vi "Map IO.vi"(8 "error in (no error)":errorcluster, 9 "Input Array":u8[](array[numeric]), 10 "Output Array":u8[](array[numeric]), 11 "6509 in":refnum<class "6509.lvclass">) -> (0 "error out":errorcluster, 1 "Boolean Array":bool[](array[boolean]), 2 "Bank Array":u8[](array[numeric]), 3 "6509 out":refnum<class "6509.lvclass">)   [LabVIEW 2019, in "6509.lvlib" / "6509.lvclass"]
uses:
  Library/6509.lvclass
  C:/Users/Public/Documents/Development/builds/Instruments/DIG_IO.lvlibp/Library/DIG_IO.lvclass
  builds/Instruments/DIG_IO.lvlibp/Accessors/Read BankDefs.vi
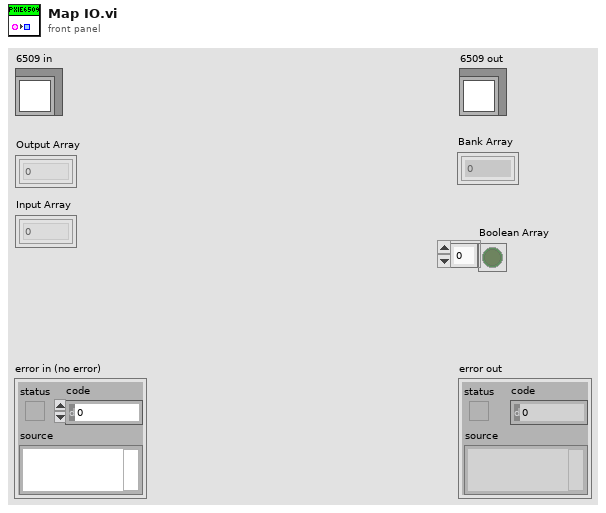
[diagram p1: front panel]
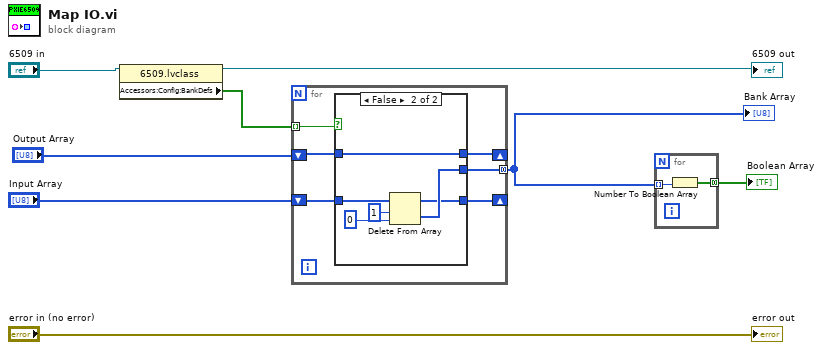
[diagram p0: block diagram]
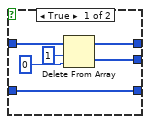
[diagram p2: hidden frame]
diagram:
  n1 = property class="6509.lvclass"(reference="6509 in") -> (reference out=→"6509 out":refnum<class "6509.lvclass">, "Accessors:Config:BankDefs"=w4:bool[])  [unwired: 1 in, 1 out]
  n2 = for {
    tunnel: w4 -> [w14] mode=indexing
    shift-right: [w10] -> _
    shift-left: "Output Array" -> [w13]
    shift-right: [w11] -> _
    shift-left: "Input Array" -> [w12]
    tunnel: [w9] -> w1 mode=concatenating
    n3 = case shown="False" w14 {
      tunnel: w13 -> [w20 w21]
      tunnel: w12 -> [w17 w23]
      tunnel: [w17 w22] -> w11
      tunnel: [w16 w21] -> w10
      tunnel: [w15 w24] -> w9
      frame True {
        n4 = Delete From Array(array=w20, length=1, index=0) -> (deleted portion=w15:u8[], array with subset deleted=w16:u8[])
      }
      frame False {
        n5 = Delete From Array(array=w23, length=1, index=0) -> (deleted portion=w24:u8[], array with subset deleted=w22:u8[])
      }
    }
  }
  "Bank Array" <- w1
  n6 = for {
    tunnel: w1 -> [w28] mode=indexing
    tunnel: [w27] -> w7 mode=concatenating
    n7 = Number To Boolean Array(number=w28) -> (Boolean array=w27:bool[])
  }
  "Boolean Array" <- w7
  "error out" <- "error in (no error)"
